vi "Conveyer Belt Move Control.vi"(1 "Conveyer Belt Information In":T1) -> (0 "Conveyer Belt Information Out":T1)   [LabVIEW 2012]
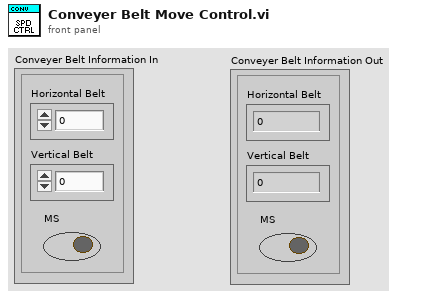
[diagram p1: front panel]
types:
  T1 = cluster{"Horizontal Belt":dbl, "Vertical Belt":dbl, "MS":bool}
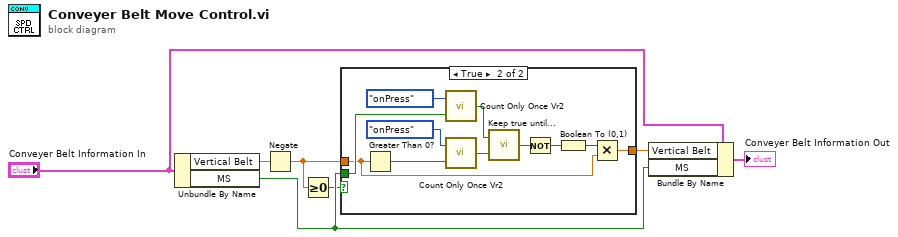
[diagram p0: block diagram]
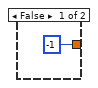
[diagram p2: hidden frame]
diagram:
  n1 = Unbundle By Name("Conveyer Belt Information In") -> ("Vertical Belt"=w3:dbl, "MS"=w4:bool)
  n2 = Negate(x=w3) -> (-x=w1:dbl)
  n3 = Greater Or Equal To 0?(x=w1) -> (x >= 0?=w2:bool)
  n4 = case shown="True" w2 {
    tunnel: [-1 w12] -> w5
    tunnel: w4 -> [_ w11]
    tunnel: w1 -> [_ w9]
    frame False {
    }
    frame True {
      n5 = Greater Than 0?(x=w9) -> (x > 0?=w10:bool)
      n6 = call "Count Only Once Vr2.vi"("InValue"=w11, "Action"=enum16{"onPress", "onRelease", "Both"}."onPress") -> ("Result"=w17:bool)
      n7 = call "Count Only Once Vr2.vi"("InValue"=w10, "Action"=enum16{"onPress", "onRelease", "Both"}."onPress") -> ("Result"=w16:bool)
      n8 = call "Keep true until....vi"("Changer"=w16, "Keep"=w17) -> ("Value"=w15:bool)
      n9 = Not(x=w15) -> (.not. x?=w14:bool)
      n10 = Boolean To (0,1)(Boolean=w14) -> (0, 1=w13:i16)
      n11 = Multiply(x=w13, y=w9) -> (x*y=w12:dbl)
    }
  }
  n12 = Bundle By Name(cluster="Conveyer Belt Information In", "Vertical Belt"=w5, "MS"=w4) -> (→"Conveyer Belt Information Out":T1)
